vi "Test Report Contain Format Definition.vi"(8 "error in (no error)":errorcluster, 11 "XML Report Test in":refnum<class "XML Report Test.lvclass">) -> (0 "error out":errorcluster, 3 "XML Report Test out":refnum<class "XML Report Test.lvclass">)   [LabVIEW 2020, in "XML Report Test.lvclass"]
uses:
  XML Report Test.lvclass
  XML Report Test.lvclass/XML Report Test.ctl
  source/Plugins/XML Report/XML Report.lvclass
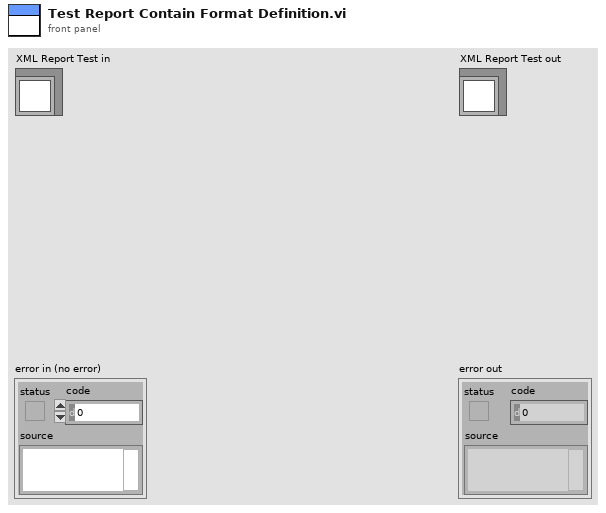
[diagram p1: front panel]
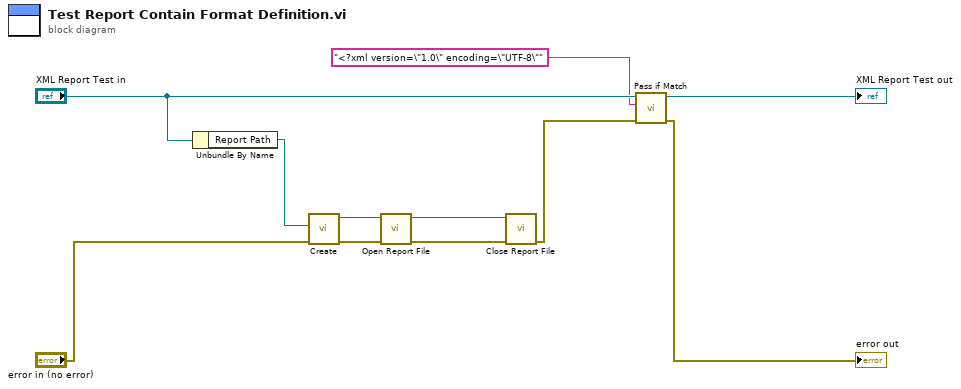
[diagram p0: block diagram]
diagram:
  n1 = Unbundle By Name("XML Report Test in") -> ("Report Path"=w2:path)
  n2 = call "Create.vi"("error in (no error)"="error in (no error)", "Report Path"=w2) -> ("error out"=w3:errorcluster, "XML Report"=w1:refnum<class "XML Report.lvclass">)  [unwired: 8 in]
  n3 = call-dynamic "Open Report File.vi"("error in (no error)"=w3, "XML Report In"=w1) -> ("error out"=w11:errorcluster, "XML Report Out"=w10:refnum<class "XML Report.lvclass">)  [unwired: 8 in]
  n4 = call-dynamic "Close Report File.vi"("error in (no error)"=w11, "XML Report In"=w10) -> ("error out"=w6:errorcluster)  [unwired: 8 in, 1 out]
  n5 = call "Pass if Match.vi"("error in (no error)"=w6, "regular expression"="<?xml version=\"1.0\" encoding=\"UTF-8\"", "XML Report Test in"="XML Report Test in") -> ("error out"=→"error out":errorcluster, "XML Report Test out"=→"XML Report Test out":refnum<class "XML Report Test.lvclass">)  [unwired: 6 in, 1 out]
